vi "Connect.vi"(6 "remote_port":u16, 7 "host_port":u16, 8 "error in (no error)":errorcluster, 9 "remote_address":string, 10 "host_address":string, 11 "Socket.Base in":refnum<class "Socket.Base.lvclass">) -> (0 "error out":errorcluster, 3 "Socket.Base out":refnum<class "Socket.Base.lvclass">)   [LabVIEW 2014, in "Socket.lvlib" / "Socket.Base.lvclass"]
doc: "(Must Be overridden) Establishes a remote connection. See the individual child classes for a description of how the input parameters are used."
uses:
  Socket.Base.lvclass
  <vilib>/Utility/error.llb/Error Cluster From Error Code.vi
  <vilib>/ErrorRing/Error Ring.xnode
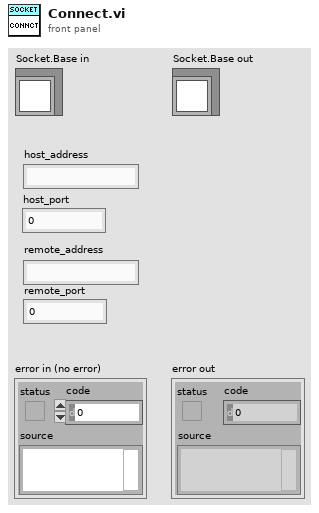
[diagram p1: front panel]
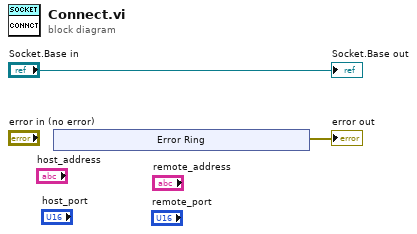
[diagram p0: block diagram]
diagram:
  n1 = xnode "Error Ring"() -> ("error out"=→"error out":errorcluster)
  "Socket.Base out" <- "Socket.Base in"
